vi "Day2.vi"(11 "Input":string) -> (3 "Result":i64)   [LabVIEW 2024]
panel:
  out "all rows":i64[][](array[numeric])
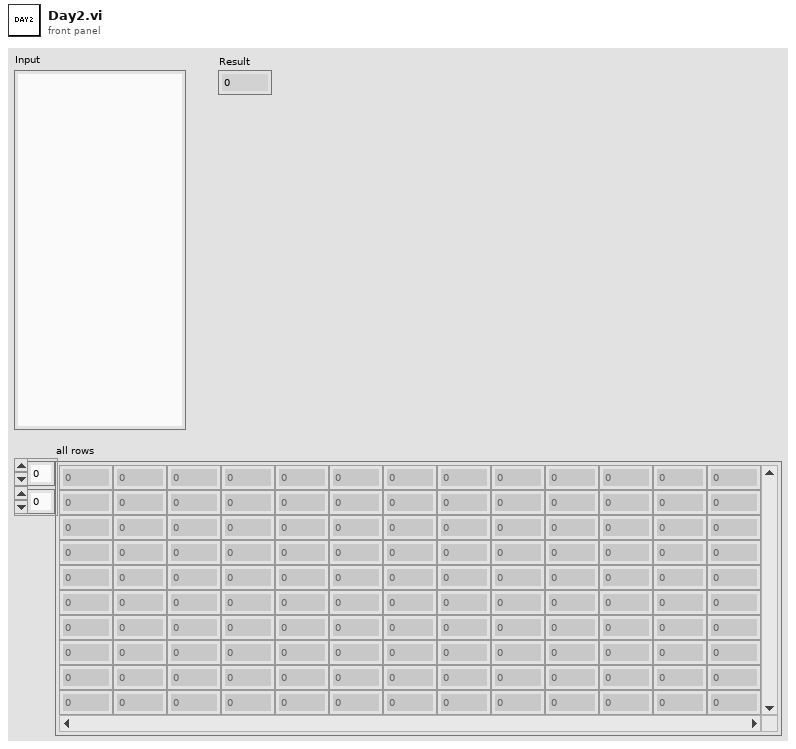
[diagram p1: front panel]
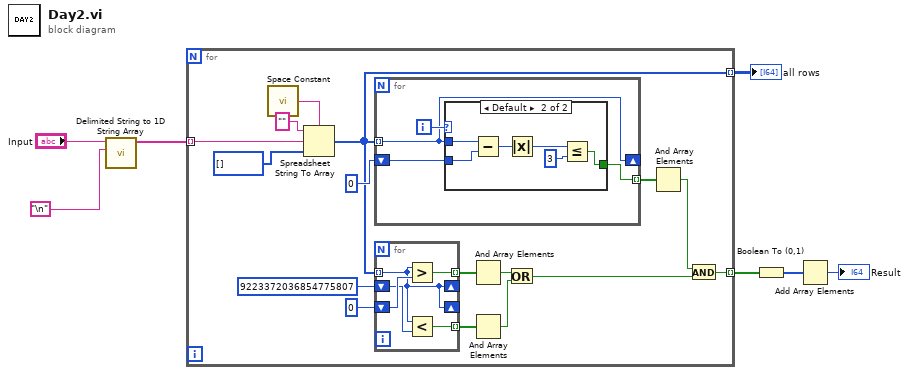
[diagram p0: block diagram]
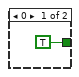
[diagram p2: hidden frame]
diagram:
  n1 = call <vilib>:"Delimited String to 1D String Array.vi"("delimiter"="\n", "delimited string"="Input") -> ("string array"=w2:string[])  [unwired: 9 in]
  n2 = for {
    tunnel: [w17] -> w6 mode=indexing
    tunnel: w2 -> [w12] mode=indexing
    tunnel: [w8] -> w4 mode=indexing
    n3 = call <vilib>:"Space Constant.vi"() -> ("String"=w9:string)
    n4 = Spreadsheet String To Array(delimiter (Tab)=w9, format string="", spreadsheet string=w12, array type (2D Dbl)=i64[] []) -> (array=w8:i64[])
    n5 = for {
      tunnel: w8 -> [w29] mode=indexing
      tunnel: [w32] -> w20 mode=indexing
      shift-right: [w29] -> _
      shift-left: i64 0 ("Numeric") -> [w31]
      i -> [w30]
      n6 = case shown="Default" w30 {
        tunnel: [TRUE w38] -> w32
        tunnel: w31 -> [_ w37]
        tunnel: w29 -> [_ w34]
        frame 0 {
        }
        frame Default {
          n7 = Subtract(x=w34, y=w37) -> (x-y=w36:i64)
          n8 = Absolute Value(x=w36) -> (abs(x)=w35:i64)
          n9 = Less Or Equal?(x=w35, y=i64 3) -> (x <= y?=w38:bool)
        }
      }
    }
    n10 = for {
      tunnel: w8 -> [w24] mode=indexing
      tunnel: [w28] -> w23 mode=indexing
      tunnel: [w27] -> w13 mode=indexing
      shift-right: [w24] -> _
      shift-left: i64 9223372036854775807 ("y") -> [w25]
      shift-right: [w24] -> _
      shift-left: i64 0 ("y") -> [w26]
      n11 = Greater?(x=w24, y=w26) -> (0:w28:bool)
      n12 = Less?(x=w24, y=w25) -> (x < y?=w27:bool)
    }
    n13 = And Array Elements(Boolean array=w23) -> (logical AND=w21:bool)
    n14 = And Array Elements(Boolean array=w13) -> (logical AND=w22:bool)
    n15 = Or(x=w21, y=w22) -> (x .or. y?=w18:bool)
    n16 = And Array Elements(Boolean array=w20) -> (logical AND=w19:bool)
    n17 = And(x=w19, y=w18) -> (x .and. y?=w17:bool)
  }
  "all rows" <- w4
  n18 = Boolean To (0,1)(Boolean=w6) -> (0, 1=w5:i16[])
  n19 = Add Array Elements(numeric array=w5) -> (sum=→"Result":i16)
